vi "Becker-Hickl Convert FLIM Dataset Info to String.vi"(5 "File Path":path, 6 "Step Duration":dbl[unit] format="%#.3g", 7 "File Size":i64, 8 "error in (no error)":errorcluster, 9 "TAC Parameters":T1, 10 "# Gates":u32, 11 "Measurement Information":T2 {"Measurement FCS Info"."FCS Type" format="%016.0f"; "Measurement FCS Info"."FCS Decay Calc" format="%016b"; "Measurement Stop Info"."Flags" format="%016b"}) -> (0 "Error Out":errorcluster, 3 "Data Description":string)   [LabVIEW 2021, in "Becker-Hickl Files.lvlib"]
uses:
  Becker-Hickl Measurement Information.ctl
  Becker-Hickl Measurement Stop Info.ctl
  Becker-Hickl FCS Measurement Info.ctl
  Becker-Hickl Additional Histogram Measurement Info.ctl
  Becker-Hickl TAC Parameters.ctl
  Becker-Hickl Files.lvlib
  Variant/Variant.lvlib
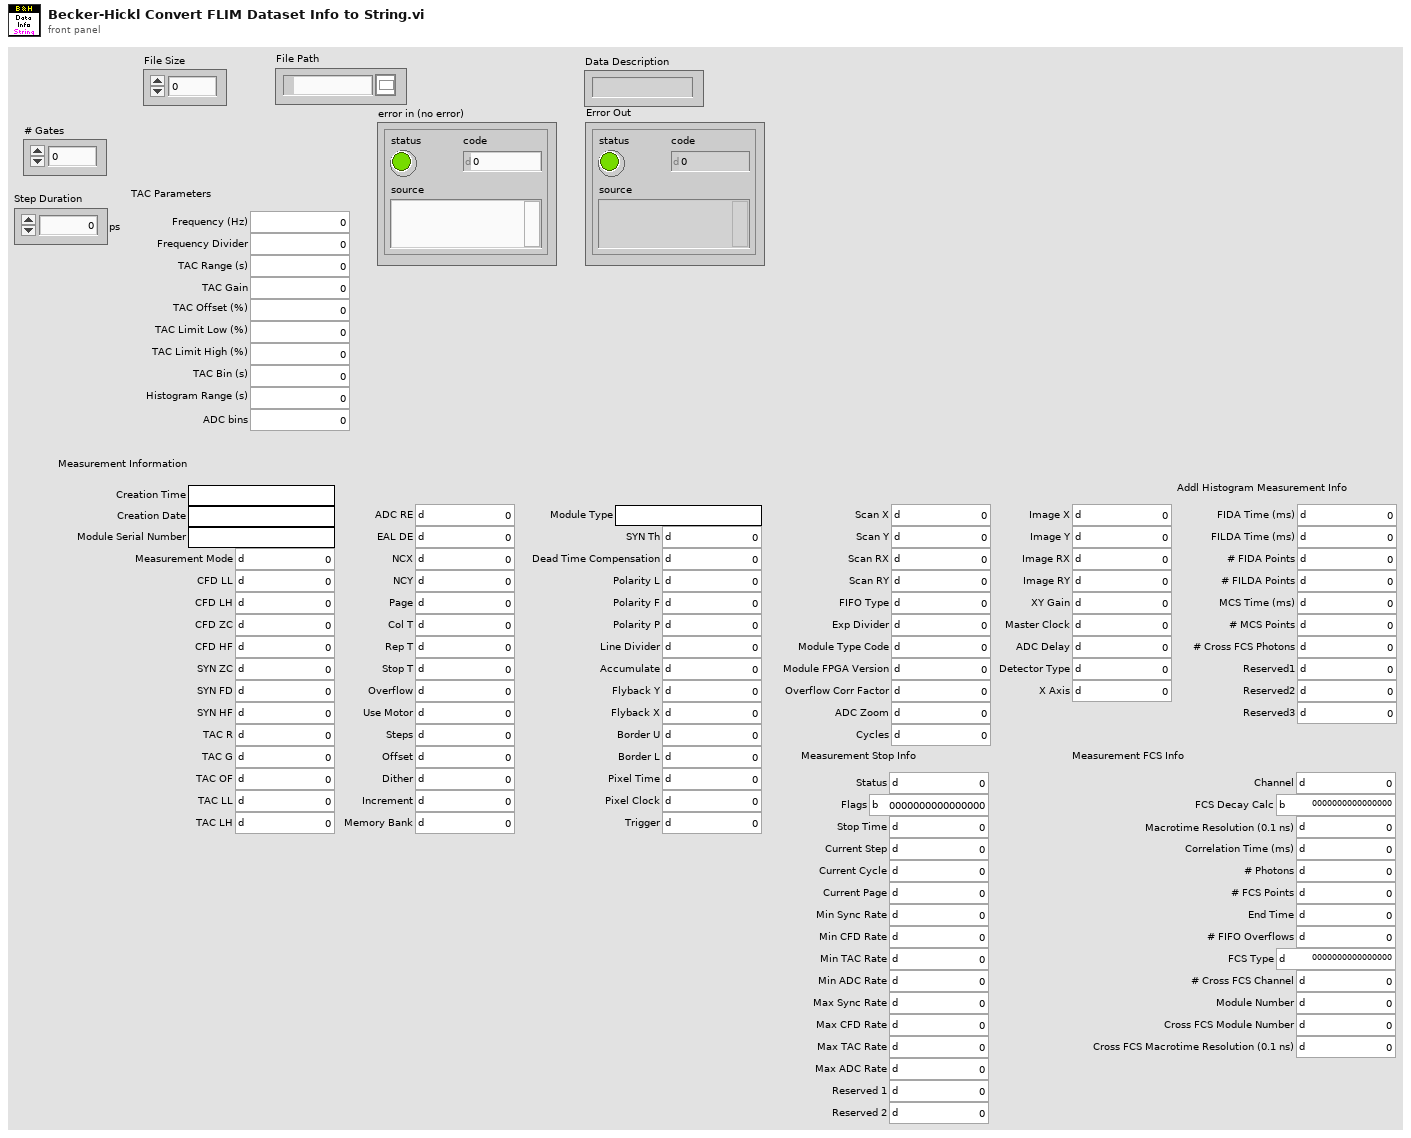
[diagram p1: front panel]
types:
  T1 = typedef "Becker-Hickl Files.lvlib/Becker-Hickl TAC Parameters.ctl" = cluster{"Frequency (Hz)":dbl, "Frequency Divider":i32, "TAC Range (s)":dbl, "TAC Gain":i32, "TAC Offset (%)":dbl, "TAC Limit Low (%)":dbl, "TAC Limit High (%)":dbl, "TAC Bin (s)":dbl, "ADC bins":i32, "Histogram Range (s)":dbl}
  T2 = typedef "Becker-Hickl Files.lvlib/Becker-Hickl Measurement Information.ctl" = cluster{"Measurement Stop Info":T3, "Measurement FCS Info":T4, "Addl Histogram Measurement Info":T5, "Creation Time":string, "Creation Date":string, "Module Serial Number":string, "Measurement Mode":i16, "CFD LL":sgl, "CFD LH":sgl, "CFD ZC":sgl, "CFD HF":sgl, "SYN ZC":sgl, "SYN FD":i16, "SYN HF":sgl, "TAC R":sgl, "TAC G":i16, "TAC OF":sgl, "TAC LL":sgl, "TAC LH":sgl, "ADC RE":i16, "EAL DE":i16, "NCX":i16, "NCY":i16, "Page":u16, "Col T":sgl, "Rep T":sgl, "Stop T":i16, "Overflow":u8, "Use Motor":i16, "Steps":u16, "Offset":sgl, "Dither":i16, "Increment":i16, "Memory Bank":i16, "Module Type":string, "SYN Th":sgl, "Dead Time Compensation":i16, "Polarity L":i16, "Polarity F":i16, "Polarity P":i16, "Line Divider":i16, "Accumulate":i16, "Flyback Y":i32, "Flyback X":i32, "Border U":i32, "Border L":i32, "Pixel Time":sgl, "Pixel Clock":i16, "Trigger":i16, "Scan X":i32, "Scan Y":i32, "Scan RX":i32, "Scan RY":i32, "FIFO Type":i16, "Exp Divider":i32, "Module Type Code":u16, "Module FPGA Version":u16, "Overflow Corr Factor":sgl, "ADC Zoom":i32, "Cycles":i32, "Image X":i32, "Image Y":i32, "Image RX":i32, "Image RY":i32, "XY Gain":i16, "Master Clock":i16, "ADC Delay":i16, "Detector Type":i16, "X Axis":i16}
  T3 = typedef "Becker-Hickl Files.lvlib/Becker-Hickl Measurement Stop Info.ctl" = cluster{"Status":u16, "Flags":u16, "Stop Time":sgl, "Current Step":i32, "Current Cycle":i32, "Current Page":i32, "Min Sync Rate":sgl, "Min CFD Rate":sgl, "Min TAC Rate":sgl, "Min ADC Rate":sgl, "Max Sync Rate":sgl, "Max CFD Rate":sgl, "Max TAC Rate":sgl, "Max ADC Rate":sgl, "Reserved 1":i32, "Reserved 2":sgl}
  T4 = typedef "Becker-Hickl Files.lvlib/Becker-Hickl FCS Measurement Info.ctl" = cluster{"Channel":u16, "FCS Decay Calc":u16, "Macrotime Resolution (0.1 ns)":u32, "Correlation Time (ms)":sgl, "# Photons":u32, "# FCS Points":i32, "End Time":sgl, "# FIFO Overflows":u16, "FCS Type":u16, "# Cross FCS Channel":u16, "Module Number":u16, "Cross FCS Module Number":u16, "Cross FCS Macrotime Resolution (0.1 ns)":u32}
  T5 = typedef "Becker-Hickl Files.lvlib/Becker-Hickl Additional Histogram Measurement Info.ctl" = cluster{"FIDA Time (ms)":sgl, "FILDA Time (ms)":sgl, "# FIDA Points":i32, "# FILDA Points":i32, "MCS Time (ms)":sgl, "# MCS Points":i32, "# Cross FCS Photons":u32, "Reserved1":i32, "Reserved2":dbl, "Reserved3":dbl}
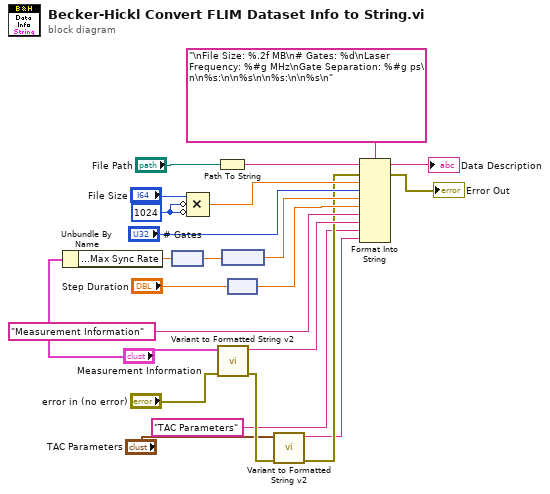
[diagram p0: block diagram]
diagram:
  w18 = i64 1024 ("y")
  n1 = Unbundle By Name("Measurement Information") -> ("Measurement Stop Info.Max Sync Rate"=w7:sgl)
  n2 = node(w7) -> (w1:sgl[unit])
  n3 = Compound Arithmetic op=MULTIPLY("File Size", invert w18, invert w18) -> (w17:dbl)
  n4 = Path To String(path="File Path") -> (string=w21:string)
  n5 = call "Variant to Formatted String v2.vi"("error in (no error)"="error in (no error)", "Anything"="Measurement Information") -> ("error out"=w6:errorcluster, "String"=w11:string)  [unwired: 8 in]
  n6 = node(w1) -> (w15:sgl)
  n7 = node("Step Duration") -> (w13:dbl)
  n8 = call "Variant to Formatted String v2.vi"("error in (no error)"=w6, "Anything"="TAC Parameters") -> ("error out"=w4:errorcluster, "String"=w2:string)  [unwired: 8 in]
  n9 = Format Into String(format string="\nFile Size: %.2f MB\n# Gates: %d\nLaser Frequency: %#g MHz\nGate Separation: %#g ps\n\n%s:\n\n%s\n\n%s:\n\n%s\n", initial string=w21, error in=w4, w17, "# Gates", w15, w13, "Measurement Information" ("Label"), w11, "TAC Parameters" ("Label"), w2) -> (resulting string=→"Data Description":string, error out=→"Error Out":errorcluster)
